vi "מסך הזמנות 8.11.vi"() -> ()   [LabVIEW 2013]
uses:
  <vilib>/Utility/file.llb/Read From Spreadsheet File (string).vi
  <vilib>/Utility/file.llb/Write To Spreadsheet File (string).vi
panel:
  in  "max":dbl
  in  "Array":dbl[](array[numeric])
  out "size(s) 2":i32[](array[numeric])
  out "number 4":i32
  out "output string 2":string
  out "decimal integer string 4":string[](array[string])
  in  "Boolean":bool
  out "String 2":string
  out "decimal integer string 3":string
  out "number 3":i32
  out "number 2":i32
  out "output string":string
  out "element 2":string
  in  "order to delete":string(combo)
  in  "Delete":bool
  in  "Cancel Button 2":bool
  in  "Compleat Order":bool
  in  "Cancel":bool
  out "x*y":dbl
  out "decimal integer string":string[](array[string])
  out "number":dbl
  out "QuantityString":string
  out "size(s)":i32[](array[numeric])
  in  "Bottle volume":string(combo)
  in  "VaccineType":string(combo)
  in  "Countru Name":string(combo)
  in  "Quantity":dbl
  out "x .or. y?":bool
  in  "String":string
  out "initialized array":string[](array[string])
  in  "Delete Order":bool
  in  "Return to":bool
  out "Fider-Order list":string[][](array[string])
  in  "Save Orders To File":bool
  in  "Create1 Order":bool
  # "Fider - Order List"
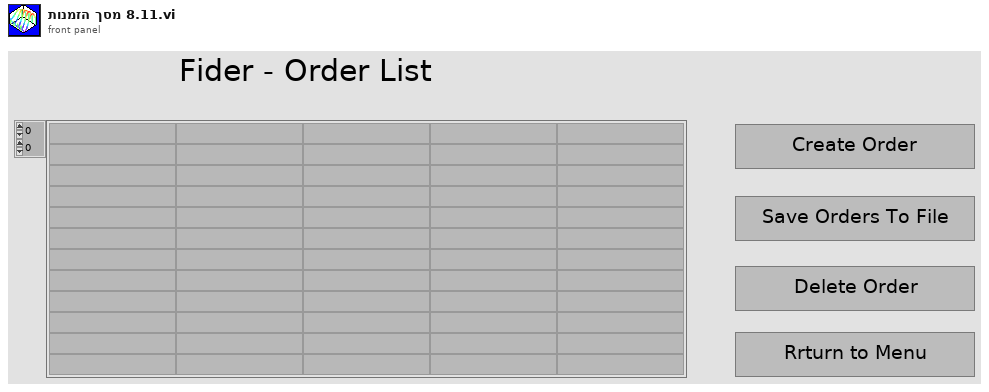
[diagram p1: front panel]
types:
  T1 = enum8{"Enabled", "Disabled", "Disabled and Grayed Out"}
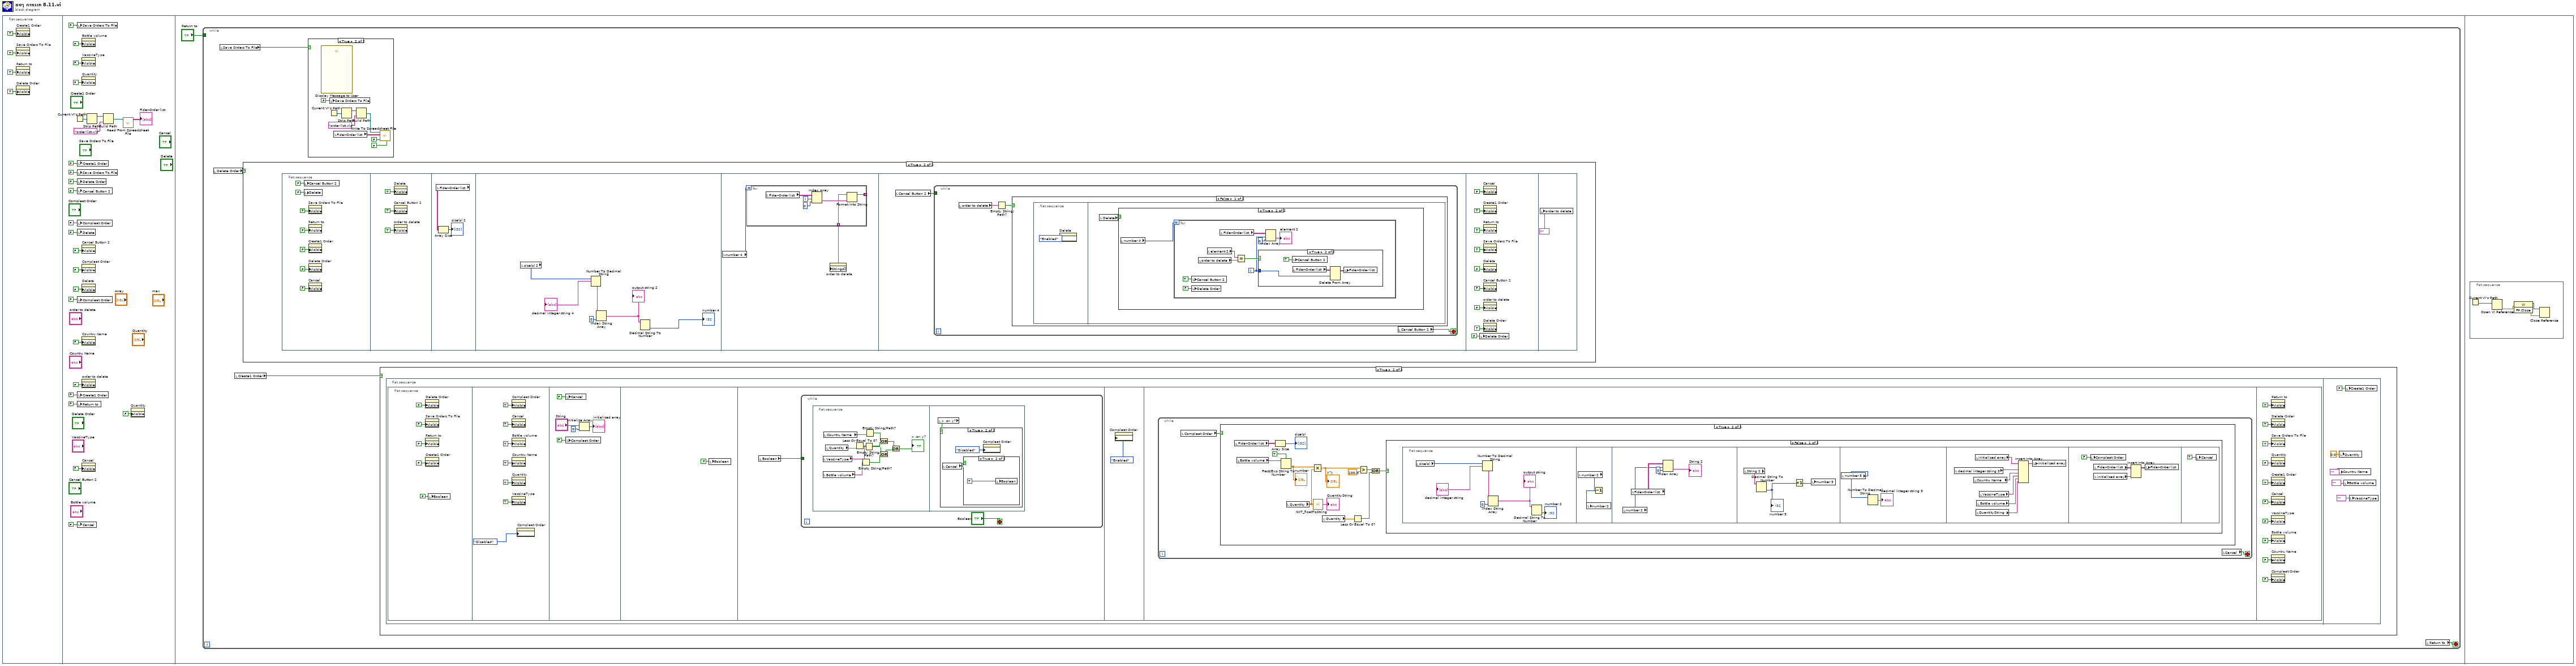
[diagram p0: block diagram]
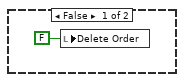
[diagram p2: hidden frame]
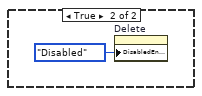
[diagram p5: hidden frame]
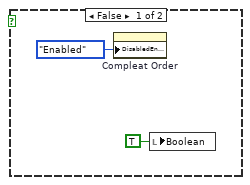
[diagram p8: hidden frame]
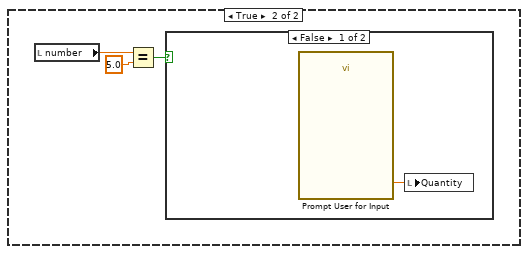
[diagram p11: hidden frame]
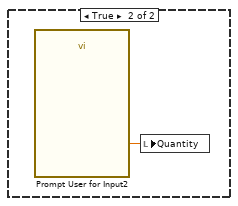
[diagram p12: hidden frame]
diagram:
  n1 = flat-sequence {
    frame #0 {
      n2 = property on="Create1 Order" class="Bool (strict)"("Visible"=TRUE) -> ()  [unwired: 2 in, 2 out]
      n3 = property on="Save Orders To File" class="Bool (strict)"("Visible"=TRUE) -> ()  [unwired: 2 in, 2 out]
      n4 = property on="Return to" class="Bool (strict)"("Visible"=TRUE) -> ()  [unwired: 2 in, 2 out]
      n5 = property on="Delete Order" class="Bool (strict)"("Visible"=TRUE) -> ()  [unwired: 2 in, 2 out]
    }
    frame #1 {
      n6 = Current VI's Path() -> (path=w27:path)
      n7 = local write "Save Orders To File"(FALSE ("Save Orders To File")) -> ()
      n8 = local write "Create1 Order"(FALSE ("Create Order")) -> ()
      n9 = local write "Save Orders To File"(FALSE ("Save Orders To File")) -> ()
      n10 = local write "Delete Order"(FALSE ("Delete Order")) -> ()
      n11 = local write "Cancel Button 2"(FALSE ("Cancel Button 2")) -> ()
      n12 = local write "Compleat Order"(FALSE ("Compleat Order")) -> ()
      n13 = local write "Delete"(FALSE ("Delete")) -> ()
      n14 = local write "Compleat Order"(FALSE ("Compleat Order")) -> ()
      n15 = local write "Create1 Order"(FALSE ("Create1 Order")) -> ()
      n16 = local write "Return to"(FALSE ("Return to")) -> ()
      n17 = local write "Cancel"(FALSE ("Cancel")) -> ()
      n18 = property on="Bottle volume" class="CmbBox"("Visible"=FALSE) -> ()  [unwired: 2 in, 2 out]
      n19 = property on="VaccineType" class="CmbBox"("Visible"=FALSE) -> ()  [unwired: 2 in, 2 out]
      n20 = property on="Quantity" class="DigNum (strict)"("Visible"=FALSE) -> ()  [unwired: 2 in, 2 out]
      n21 = property on="Cancel Button 2" class="Bool (strict)"("Visible"=FALSE) -> ()  [unwired: 2 in, 2 out]
      n22 = property on="Compleat Order" class="Bool (strict)"("Visible"=FALSE) -> ()  [unwired: 2 in, 2 out]
      n23 = property on="Delete" class="Bool (strict)"("Visible"=FALSE) -> ()  [unwired: 2 in, 2 out]
      n24 = property on="Countru Name" class="CmbBox"("Visible"=FALSE) -> ()  [unwired: 2 in, 2 out]
      n25 = property on="order to delete" class="CmbBox"("Visible"=FALSE) -> ()  [unwired: 2 in, 2 out]
      n26 = property on="Cancel" class="Bool (strict)"("Visible"=FALSE) -> ()  [unwired: 2 in, 2 out]
      n27 = Strip Path(path=w27) -> (stripped path=w28:path)  [unwired: 1 out]
      n28 = Build Path(base path=w28, name or relative path="order list.xls") -> (appended path=w26:path)
      n29 = call-poly <vilib>:"Read From Spreadsheet File.vi"("file path (dialog if empty)"=w26) -> ("all rows"=→"Fider-Order list":string[][])  [unwired: 6 in, 4 out]
      n30 = property on="Quantity" class="DigNum (strict)"("Visible"=FALSE) -> ()  [unwired: 2 in, 2 out]
    }
    frame #2 {
      n31 = while {
        tunnel: "Return to" -> [_]
        stop <- w35 stop-if-true
        n32 = local read "Delete Order"() -> (w33:bool)
        n33 = local read "Save Orders To File"() -> (w32:bool)
        n34 = local read "Create1 Order"() -> (w34:bool)
        n35 = case shown="True" w33 {
          frame False {
            n36 = local write "Delete Order"(FALSE ("Delete Order")) -> ()
          }
          frame True {
            n37 = flat-sequence {
              frame #0 {
                n38 = local write "Cancel Button 2"(FALSE ("Cancel Button 2")) -> ()
                n39 = local write "Delete"(FALSE ("Delete")) -> ()
                n40 = property on="Save Orders To File" class="Bool (strict)"("Visible"=FALSE) -> ()  [unwired: 2 in, 2 out]
                n41 = property on="Return to" class="Bool (strict)"("Visible"=FALSE) -> ()  [unwired: 2 in, 2 out]
                n42 = property on="Create1 Order" class="Bool (strict)"("Visible"=FALSE) -> ()  [unwired: 2 in, 2 out]
                n43 = property on="Delete Order" class="Bool (strict)"("Visible"=FALSE) -> ()  [unwired: 2 in, 2 out]
                n44 = property on="Cancel" class="Bool (strict)"("Visible"=FALSE) -> ()  [unwired: 2 in, 2 out]
              }
              frame #1 {
                n45 = property on="Delete" class="Bool (strict)"("Visible"=TRUE) -> ()  [unwired: 2 in, 2 out]
                n46 = property on="Cancel Button 2" class="Bool (strict)"("Visible"=TRUE) -> ()  [unwired: 2 in, 2 out]
                n47 = property on="order to delete" class="CmbBox"("Visible"=TRUE) -> ()  [unwired: 2 in, 2 out]
              }
              frame #2 {
                n48 = local read "Fider-Order list"() -> (w48:string[][])
                n49 = Array Size(array=w48) -> (size(s)=→"size(s) 2":i32[])
              }
              frame #3 {
                n50 = local read "size(s) 2"() -> (w49:i32[])
                n51 = Number To Decimal String(number=w49) -> (decimal integer string=w51:string[])  [unwired: 1 in]
                "decimal integer string 4" <- w51
                n52 = Index String Array(1:0 ("index"), 2:w51) -> (0:w52:string)  [unwired: 1 in]
                "output string 2" <- w52
                n53 = Decimal String To Number(string=w52) -> (number=→"number 4":i32)  [unwired: 2 in, 1 out]
              }
              frame #4 {
                n54 = local read "number 4"() -> (w54:i32)
                n55 = for {
                  N: w54 -> [_]
                  tunnel: [w56] -> _ mode=indexing
                  tunnel: [w56] -> w55 mode=indexing
                  i -> [w59]
                  n56 = local read "Fider-Order list"() -> (w57:string[][])
                  n57 = Index Array(array=w57, index (row)=w59, index (col)=0 ("disabled index (col)")) -> (element=w58:string)
                  n58 = Format Into String(w58) -> (resulting string=w56:string)  [unwired: 3 in, 1 out]
                }
                n59 = property on="order to delete" class="CmbBox"("Strings[]"=w55) -> ()  [unwired: 2 in, 2 out]
              }
              frame #5 {
                n60 = local read "Cancel Button 2"() -> (w61:bool)
                n61 = while {
                  tunnel: w61 -> [_]
                  stop <- w64 stop-if-true
                  n62 = local read "order to delete"() -> (w63:string)
                  n63 = Empty String/Path?(string/path=w63) -> (empty?=w62:bool)
                  n64 = case shown="False" w62 {
                    frame False {
                      n65 = flat-sequence {
                        frame #0 {
                          n66 = property on="Delete" class="Bool (strict)"("DisabledEnum"=T1."Enabled" ("Disabled")) -> ()  [unwired: 2 in, 2 out]
                        }
                        frame #1 {
                          n67 = local read "Delete"() -> (w66:bool)
                          n68 = case shown="True" w66 {
                            frame False {
                            }
                            frame True {
                              n69 = local read "number 4"() -> (w67:i32)
                              n70 = for {
                                N: w67 -> [_]
                                i -> [w70]
                                n71 = local write "Cancel Button 2"(TRUE ("Cancel Button 2")) -> ()
                                n72 = local write "Delete Order"(FALSE ("Delete Order")) -> ()
                                n73 = local read "order to delete"() -> (w74:string)
                                n74 = local read "element 2"() -> (w73:string)
                                n75 = local read "Fider-Order list"() -> (w75:string[][])
                                n76 = Equal?(x=w73, y=w74) -> (x = y?=w72:bool)
                                n77 = case shown="True" w72 {
                                tunnel: w70 -> [_ w77]
                                frame False {
                                }
                                frame True {
                                n78 = local write "Cancel Button 2"(TRUE ("Cancel Button 2")) -> ()
                                n79 = local read "Fider-Order list"() -> (w79:string[][])
                                n80 = Delete From Array(array=w79, index (row)=w77) -> (array with subset deleted=w78:string[][])  [unwired: 2 in, 1 out]
                                n81 = local write "Fider-Order list"(w78) -> ()
                                }
                                }
                                n82 = Index Array(array=w75, index (row)=w70, index (col)=0 ("disabled index (col)")) -> (element=→"element 2":string)
                              }
                            }
                          }
                        }
                      }
                    }
                    frame True {
                      n83 = property on="Delete" class="Bool (strict)"("DisabledEnum"=T1."Disabled" ("Disabled")) -> ()  [unwired: 2 in, 2 out]
                    }
                  }
                  n84 = local read "Cancel Button 2"() -> (w64:bool)
                }
              }
              frame #6 {
                n85 = local write "Delete Order"(FALSE ("Delete Order")) -> ()
                n86 = property on="Cancel" class="Bool (strict)"("Visible"=FALSE) -> ()  [unwired: 2 in, 2 out]
                n87 = property on="Create1 Order" class="Bool (strict)"("Visible"=TRUE) -> ()  [unwired: 2 in, 2 out]
                n88 = property on="Return to" class="Bool (strict)"("Visible"=TRUE) -> ()  [unwired: 2 in, 2 out]
                n89 = property on="Save Orders To File" class="Bool (strict)"("Visible"=TRUE) -> ()  [unwired: 2 in, 2 out]
                n90 = property on="Delete" class="Bool (strict)"("Visible"=FALSE) -> ()  [unwired: 2 in, 2 out]
                n91 = property on="Cancel Button 2" class="Bool (strict)"("Visible"=FALSE) -> ()  [unwired: 2 in, 2 out]
                n92 = property on="order to delete" class="CmbBox"("Visible"=FALSE) -> ()  [unwired: 2 in, 2 out]
                n93 = property on="Delete Order" class="Bool (strict)"("Visible"=TRUE) -> ()  [unwired: 2 in, 2 out]
              }
              frame #7 {
                n94 = local write "order to delete"("" ("oeder to delete")) -> ()
              }
            }
          }
        }
        n95 = case shown="True" w32 {
          frame False {
          }
          frame True {
            n96 = call "Display Message to User"() -> ()  [unwired: 10 in, 2 out]
            n97 = Current VI's Path() -> (path=w99:path)
            n98 = local write "Save Orders To File"(FALSE ("Save Orders To File")) -> ()
            n99 = local read "Fider-Order list"() -> (w96:string[][])
            n100 = Strip Path(path=w99) -> (stripped path=w98:path)  [unwired: 1 out]
            n101 = Build Path(base path=w98, name or relative path="order list.xls") -> (appended path=w97:path)
            n102 = call-poly <vilib>:"Write To Spreadsheet File.vi"("transpose? (no:F)"=FALSE, "append to file? (new file:F)"=FALSE, "2D data"=w96, "file path (dialog if empty)"=w97) -> ()  [unwired: 4 in, 1 out]
          }
        }
        n103 = case shown="True" w34 {
          frame False {
          }
          frame True {
            n104 = flat-sequence {
              frame #0 {
                n105 = flat-sequence {
                  frame #0 {
                    n106 = property on="Delete Order" class="Bool (strict)"("Visible"=FALSE) -> ()  [unwired: 2 in, 2 out]
                    n107 = property on="Save Orders To File" class="Bool (strict)"("Visible"=FALSE) -> ()  [unwired: 2 in, 2 out]
                    n108 = property on="Return to" class="Bool (strict)"("Visible"=FALSE) -> ()  [unwired: 2 in, 2 out]
                    n109 = property on="Create1 Order" class="Bool (strict)"("Visible"=FALSE) -> ()  [unwired: 2 in, 2 out]
                    n110 = local write "Boolean"(FALSE ("Boolean")) -> ()
                  }
                  frame #1 {
                    n111 = property on="Compleat Order" class="Bool (strict)"("Visible"=TRUE) -> ()  [unwired: 2 in, 2 out]
                    n112 = property on="Cancel" class="Bool (strict)"("Visible"=TRUE) -> ()  [unwired: 2 in, 2 out]
                    n113 = property on="Bottle volume" class="CmbBox"("Visible"=TRUE) -> ()  [unwired: 2 in, 2 out]
                    n114 = property on="Countru Name" class="CmbBox"("Visible"=TRUE) -> ()  [unwired: 2 in, 2 out]
                    n115 = property on="Quantity" class="DigNum (strict)"("Visible"=TRUE) -> ()  [unwired: 2 in, 2 out]
                    n116 = property on="VaccineType" class="CmbBox"("Visible"=TRUE) -> ()  [unwired: 2 in, 2 out]
                    n117 = property on="Compleat Order" class="Bool (strict)"("DisabledEnum"=T1."Disabled" ("Disabled")) -> ()  [unwired: 2 in, 2 out]
                  }
                  frame #2 {
                    n118 = local write "Cancel"(FALSE ("Cancel")) -> ()
                    n119 = local write "Compleat Order"(FALSE ("Compleat Order")) -> ()
                    n120 = Initialize Array("String", 0 ("dimension size")) -> (→"initialized array":string[])
                  }
                  frame #3 {
                    n121 = local write "Boolean"(FALSE ("Boolean")) -> ()
                  }
                  frame #4 {
                    n122 = local read "Boolean"() -> (w118:bool)
                    n123 = while {
                      tunnel: w118 -> [_]
                      stop <- "Boolean" stop-if-true
                      n124 = flat-sequence {
                        frame #0 {
                          n125 = local read "VaccineType"() -> (w129:string)
                          n126 = local read "Bottle volume"() -> (w128:string)
                          n127 = local read "Countru Name"() -> (w130:string)
                          n128 = local read "Quantity"() -> (w127:dbl)
                          n129 = Less Or Equal To 0?(x=w127) -> (x <= 0?=w124:bool)
                          n130 = Empty String/Path?(string/path=w128) -> (empty?=w123:bool)
                          n131 = Empty String/Path?(string/path=w129) -> (empty?=w125:bool)
                          n132 = Empty String/Path?(string/path=w130) -> (empty?=w126:bool)
                          n133 = Or(x=w124, y=w123) -> (x .or. y?=w121:bool)
                          n134 = Or(x=w126, y=w125) -> (x .or. y?=w122:bool)
                          n135 = Or(x=w122, y=w121) -> (x .or. y?=→"x .or. y?":bool)
                        }
                        frame #1 {
                          n136 = local read "x .or. y?"() -> (w131:bool)
                          n137 = case shown="True" w131 {
                            frame False {
                              n138 = property on="Compleat Order" class="Bool (strict)"("DisabledEnum"=T1."Enabled" ("Disabled")) -> ()  [unwired: 2 in, 2 out]
                              n139 = local write "Boolean"(TRUE ("Boolean")) -> ()
                            }
                            frame True {
                              n140 = local read "Cancel"() -> (w134:bool)
                              n141 = case shown="True" w134 {
                                frame False {
                                }
                                frame True {
                                n142 = local write "Boolean"(TRUE ("Boolean")) -> ()
                                }
                              }
                              n143 = property on="Compleat Order" class="Bool (strict)"("DisabledEnum"=T1."Disabled" ("Disabled")) -> ()  [unwired: 2 in, 2 out]
                            }
                          }
                        }
                      }
                    }
                  }
                  frame #5 {
                    n144 = property on="Compleat Order" class="Bool (strict)"("DisabledEnum"=T1."Enabled" ("Disabled")) -> ()  [unwired: 2 in, 2 out]
                  }
                  frame #6 {
                    n145 = while {
                      stop <- w138 stop-if-true
                      n146 = local read "Compleat Order"() -> (w139:bool)
                      n147 = case shown="True" w139 {
                        frame False {
                        }
                        frame True {
                          n148 = local read "Fider-Order list"() -> (w140:string[][])
                          n149 = local read "Bottle volume"() -> (w150:string)
                          n150 = Array Size(array=w140) -> (size(s)=→"size(s)":i32[])
                          n151 = Fract/Exp String To Number(use system decimal point (T)=TRUE, string=w150) -> (number=w148:dbl)  [unwired: 2 in, 1 out]
                          "number" <- w148
                          n152 = local read "Quantity"() -> (w146:dbl)
                          n153 = Multiply(x=w148, y=w146) -> (x*y=w152:dbl)
                          "x*y" <- w152
                          n154 = call <vilib>:"NXT_floatToString.vi"("number"=w146) -> ("string"=→"QuantityString":string)
                          n155 = local read "Quantity"() -> (w145:dbl)
                          n156 = Less Or Equal To 0?(x=w145) -> (x <= 0?=w143:bool)
                          n157 = Greater?(x=w152, y=100.0) -> (0:w144:bool)
                          n158 = Or(x=w144, y=w143) -> (x .or. y?=w142:bool)
                          n159 = case shown="False" w142 {
                            frame False {
                              n160 = flat-sequence {
                                frame #0 {
                                n161 = local read "size(s)"() -> (w153:i32[])
                                n162 = Number To Decimal String(number=w153) -> (decimal integer string=w155:string[])  [unwired: 1 in]
                                "decimal integer string" <- w155
                                n163 = Index String Array(1:0 ("index"), 2:w155) -> (0:w156:string)  [unwired: 1 in]
                                "output string" <- w156
                                n164 = Decimal String To Number(string=w156) -> (number=→"number 2":i32)  [unwired: 2 in, 1 out]
                                }
                                frame #1 {
                                n165 = local read "number 2"() -> (w159:i32)
                                n166 = Decrement(x=w159) -> (x-1=w158:i32)
                                n167 = local write "number 2"(w158) -> ()
                                }
                                frame #2 {
                                n168 = local read "number 2"() -> (w162:i32)
                                n169 = local read "Fider-Order list"() -> (w163:string[][])
                                n170 = Index Array(array=w163, index (row)=w162, index (col)=0 ("disabled index (col)")) -> (element=→"String 2":string)
                                }
                                frame #3 {
                                n171 = local read "String 2"() -> (w164:string)
                                n172 = Decimal String To Number(string=w164) -> (number=w166:i32)  [unwired: 2 in, 1 out]
                                "number 3" <- w166
                                n173 = Increment(x=w166) -> (x+1=w165:i32)
                                n174 = local write "number 3"(w165) -> ()
                                }
                                frame #4 {
                                n175 = local read "number 3"() -> (w168:i32)
                                n176 = Number To Decimal String(number=w168) -> (decimal integer string=→"decimal integer string 3":string)  [unwired: 1 in]
                                }
                                frame #5 {
                                n177 = local read "decimal integer string 3"() -> (w169:string)
                                n178 = local read "Countru Name"() -> (w175:string)
                                n179 = local read "initialized array"() -> (w171:string[])
                                n180 = local read "QuantityString"() -> (w172:string)
                                n181 = local read "Bottle volume"() -> (w173:string)
                                n182 = local read "VaccineType"() -> (w174:string)
                                n183 = Insert Into Array(array=w171, new element #1=w169, new element #2=w175, new element #3=w174, new element #4=w173, new element #5=w172) -> (w170:string[])  [unwired: 1 in]
                                n184 = local write "initialized array"(w170) -> ()
                                }
                                frame #6 {
                                n185 = local write "Compleat Order"(FALSE ("Compleat Order")) -> ()
                                n186 = local read "Fider-Order list"() -> (w177:string[][])
                                n187 = local read "initialized array"() -> (w179:string[])
                                n188 = Insert Into Array(array=w177, new element=w179) -> (w178:string[][])  [unwired: 2 in]
                                n189 = local write "Fider-Order list"(w178) -> ()
                                }
                                frame #7 {
                                n190 = local write "Cancel"(TRUE ("Cancel")) -> ()
                                }
                              }
                            }
                            frame True {
                              n191 = local read "number"() -> (w183:dbl)
                              n192 = Equal?(x=w183, y=5.0) -> (x = y?=w181:bool)
                              n193 = case shown="False" w181 {
                                frame False {
                                n194 = call "Prompt User for Input"() -> ("Quantity"=w184:dbl)  [unwired: 17 in, 2 out]
                                n195 = local write "Quantity"(w184) -> ()
                                }
                                frame True {
                                n196 = call "Prompt User for Input2"() -> ("Quantity"=w185:dbl)  [unwired: 17 in, 2 out]
                                n197 = local write "Quantity"(w185) -> ()
                                }
                              }
                            }
                          }
                        }
                      }
                      n198 = local read "Cancel"() -> (w138:bool)
                    }
                  }
                  frame #7 {
                    n199 = property on="Return to" class="Bool (strict)"("Visible"=TRUE) -> ()  [unwired: 2 in, 2 out]
                    n200 = property on="Delete Order" class="Bool (strict)"("Visible"=TRUE) -> ()  [unwired: 2 in, 2 out]
                    n201 = property on="Save Orders To File" class="Bool (strict)"("Visible"=TRUE) -> ()  [unwired: 2 in, 2 out]
                    n202 = property on="Quantity" class="DigNum (strict)"("Visible"=FALSE) -> ()  [unwired: 2 in, 2 out]
                    n203 = property on="Create1 Order" class="Bool (strict)"("Visible"=TRUE) -> ()  [unwired: 2 in, 2 out]
                    n204 = property on="Cancel" class="Bool (strict)"("Visible"=FALSE) -> ()  [unwired: 2 in, 2 out]
                    n205 = property on="VaccineType" class="CmbBox"("Visible"=FALSE) -> ()  [unwired: 2 in, 2 out]
                    n206 = property on="Bottle volume" class="CmbBox"("Visible"=FALSE) -> ()  [unwired: 2 in, 2 out]
                    n207 = property on="Countru Name" class="CmbBox"("Visible"=FALSE) -> ()  [unwired: 2 in, 2 out]
                    n208 = property on="Compleat Order" class="Bool (strict)"("Visible"=FALSE) -> ()  [unwired: 2 in, 2 out]
                  }
                }
              }
              frame #1 {
                n209 = local write "Countru Name"("" ("Countru Name")) -> ()
                n210 = local write "Quantity"(0.0 ("Quantity")) -> ()
                n211 = local write "Bottle volume"("" ("Bottle volume")) -> ()
                n212 = local write "Create1 Order"(FALSE ("Create Order")) -> ()
                n213 = local write "VaccineType"("" ("VaccineType")) -> ()
              }
            }
          }
        }
        n214 = local read "Return to"() -> (w35:bool)
      }
    }
    frame #3 {
      n215 = flat-sequence {
        frame #0 {
          n216 = Current VI's Path() -> (path=w204:path)
          n217 = Open VI Reference(vi path=w204) -> (error out=w203:errorcluster)  [unwired: 5 in, 1 out]
          n218 = invoke class="VI" method="FP.Close"(error in=w203) -> (reference out=w201:refnum<vi>, error out=w202:errorcluster)  [unwired: 2 in, 1 out]
          n219 = Close Reference(reference=w201, error in (no error)=w202) -> ()  [unwired: 1 out]
        }
      }
    }
  }
